vi "OB Init.vi"(9 "EnInternalPull":u8, 10 "Channel":u8, 11 "DevHandle":i32) -> (3 "function return":i32)   [LabVIEW 2010, in "usb2openbus.lvlib"]
doc: "int WINAPI OB_Init(int DevHandle, unsigned char Channel,unsigned char EnInternalPull);"
uses:
  usb2openbus.lvlib
  USB2XXX.dll
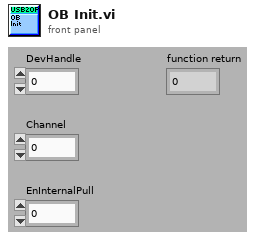
[diagram p1: front panel]
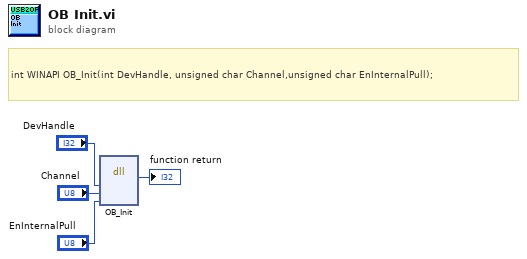
[diagram p0: block diagram]
diagram:
  # "int WINAPI OB_Init(int DevHandle, unsigned char Channel,unsigned char EnInternalPull);"
  n1 = dll-call lib="F:/OtherWork/STM32/USB2XXX_Example/trunk/Labview/PublicFiles/usb2openbus/USB2XXX.*" fn="OB_Init"("DevHandle"="DevHandle", "Channel"="Channel", "EnInternalPull"="EnInternalPull") -> (→"function return":i32)  [unwired: 6 in, 2 out]
